vi "Collide.vi"(8 "error in (no error)":errorcluster, 9 "angleCorrection in":sgl, 10 "action in":T1, 11 "class data in":refnum<class "SceneObject.lvclass">) -> (0 "error out":errorcluster, 3 "class data out":refnum<class "SceneObject.lvclass">)   [LabVIEW 2010, in "RenderBase.lvlib" / "SceneObject.lvclass"]
doc: "Callback method that is run on collision. This is not an abstract method but a default implementation that does nothing (not every scene object might need a collision check). It must be overridden by a child class to implement a particular collision check."
uses:
  SceneObject.lvclass
  CollisionAction.ctl
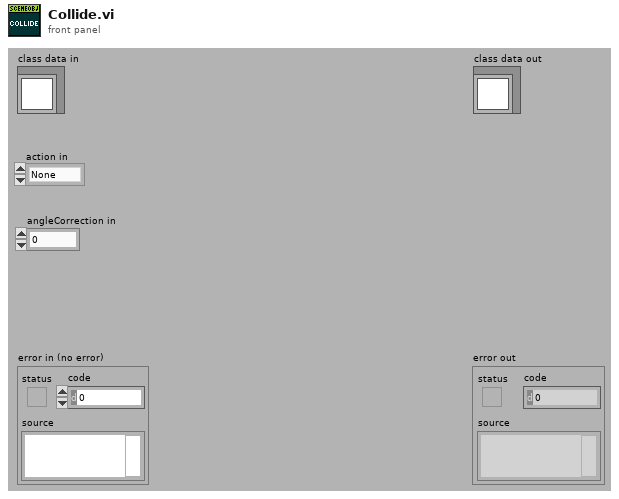
[diagram p1: front panel]
types:
  T1 = typedef "RenderBase.lvlib/SceneObject.lvclass/CollisionAction.ctl" = enum16{"None", "BounceX", "BounceY", "BounceXY"}
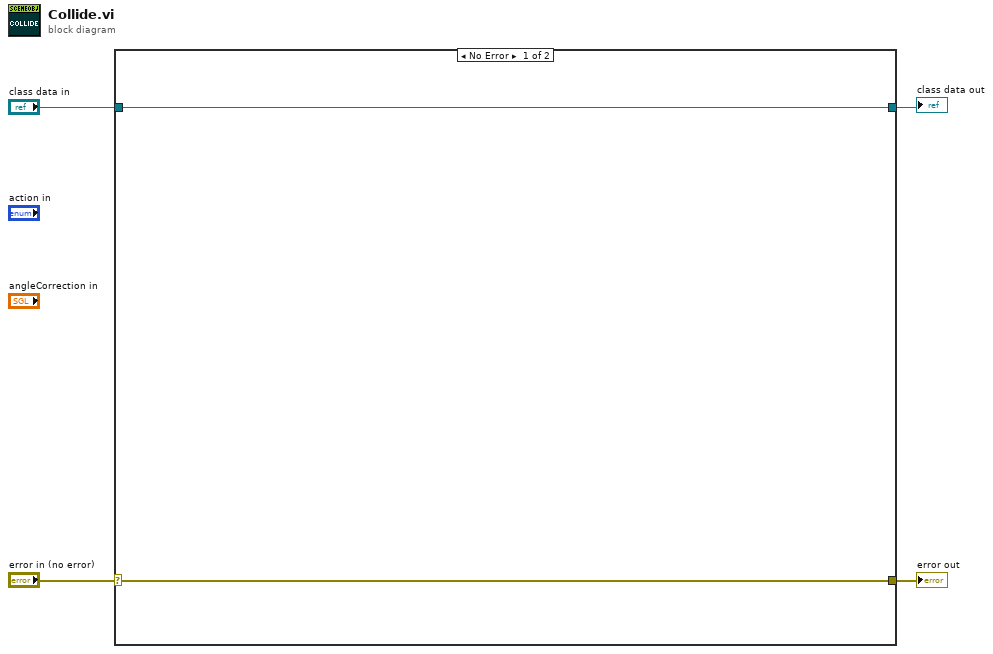
[diagram p0: block diagram]
diagram:
  n1 = case shown="No Error" "error in (no error)" {
    selector: "error in (no error)" -> [w6 w8]
    tunnel: [w6 w8] -> w3
    tunnel: "class data in" -> [w5 w7]
    tunnel: [w5 w7] -> w1
    frame No Error {
    }
    frame Error {
    }
  }
  "error out" <- w3
  "class data out" <- w1
